vi "MLUG_Item_OnCommand.vi"(10 "Command ID":string, 11 "Object":T1) -> ()   [LabVIEW 2020]
uses:
  <resource>/Framework/Providers/API/ItemRef.ctl
panel:
  out "error out":errorcluster
  in  "error in":errorcluster
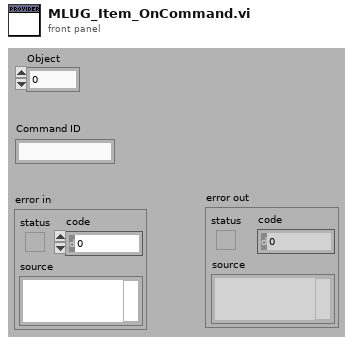
[diagram p1: front panel]
types:
  T1 = typedef "ItemRef.ctl" = u64
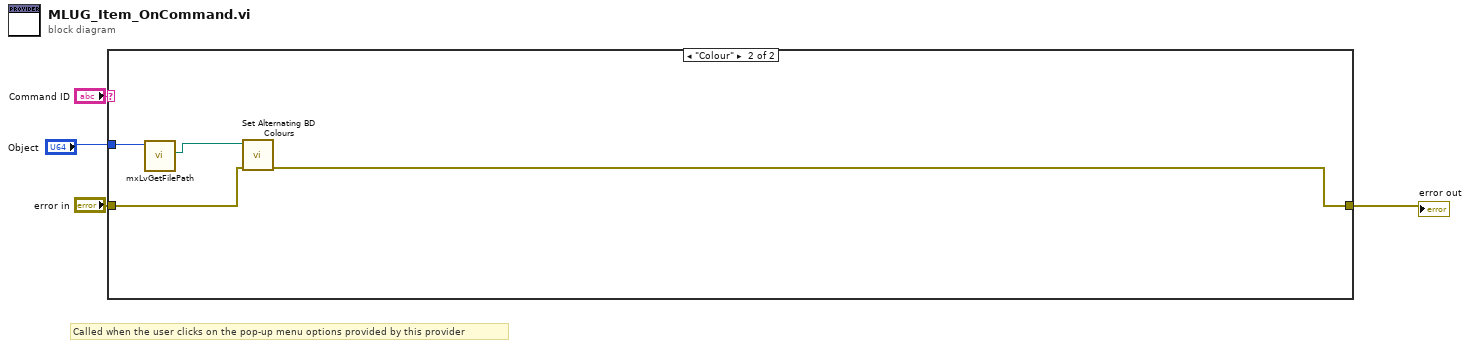
[diagram p0: block diagram]
diagram:
  # "Called when the user clicks on the pop-up menu options provided by this provider"
  n1 = case shown="\"Colour\"" "Command ID" {
    tunnel: "error in" -> [w5 w7]
    tunnel: [w5 w6] -> w2
    tunnel: "Object" -> [_ w9]
    frame Default {
    }
    frame "Colour" {
      n2 = call <resource>:"mxLvGetFilePath.vi"("Item"=w9) -> ("File Path"=w8:path)  [unwired: 8 in, 2 out]
      n3 = call <resource>:"Set Alternating BD Colours.vi"("error in (no error)"=w7, "VI Path"=w8) -> ("error out"=w6:errorcluster)  [unwired: 9 in]
    }
  }
  "error out" <- w2
